vi "TCL.vi"() -> ()   [LabVIEW 2010]
uses:
  TPS Global.vi
panel:
  out "discarded fragments":string[](array[string])
  out "signals":cluster{"name":string, "values":string[]}[](array[cluster])
  out "events (last 11)":string[][](array[string])
  out "fragments":string[](array[string])
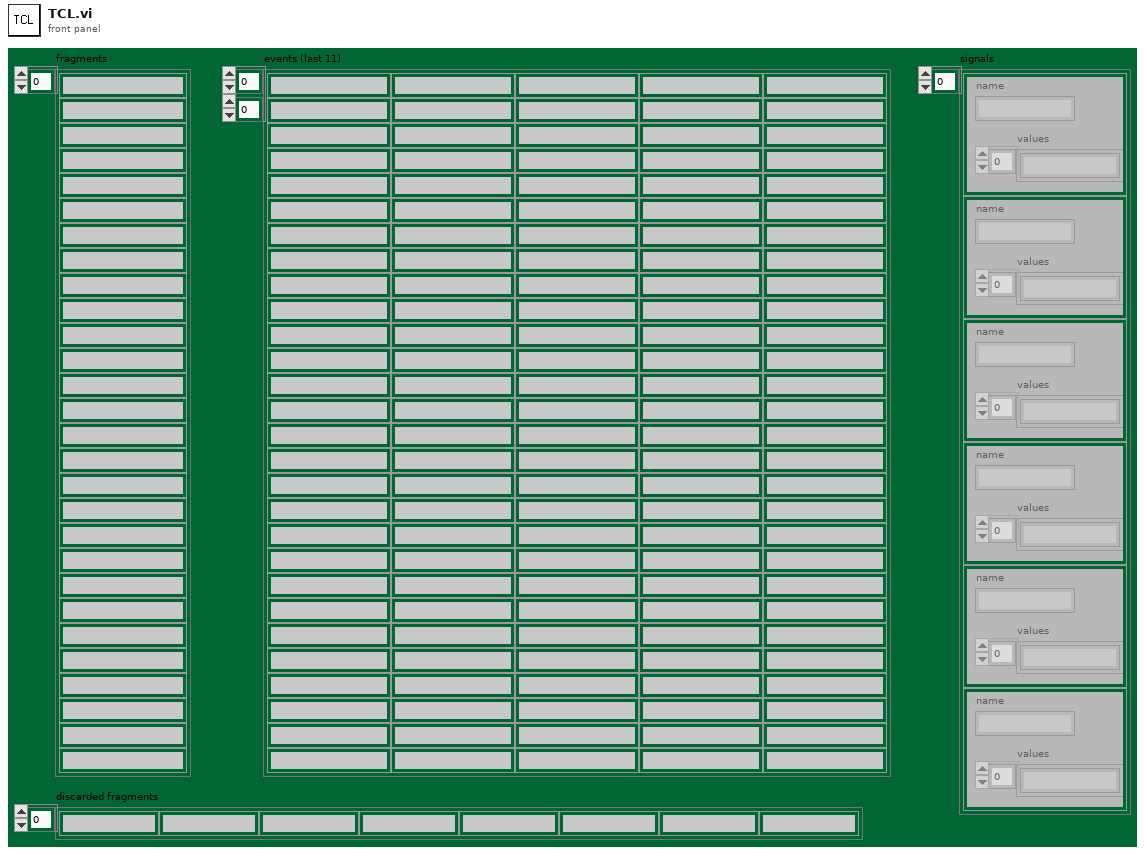
[diagram p1: front panel]
types:
  T1 = enum16{"open", "replace", "create", "open or create", "replace or create", "replace or create with confirmation"}
  T2 = enum16{"No Message", "Bad Message", "NewEventFile", "NewBaseFile", "Event=", "Ping=", "Address=", "Stop"}
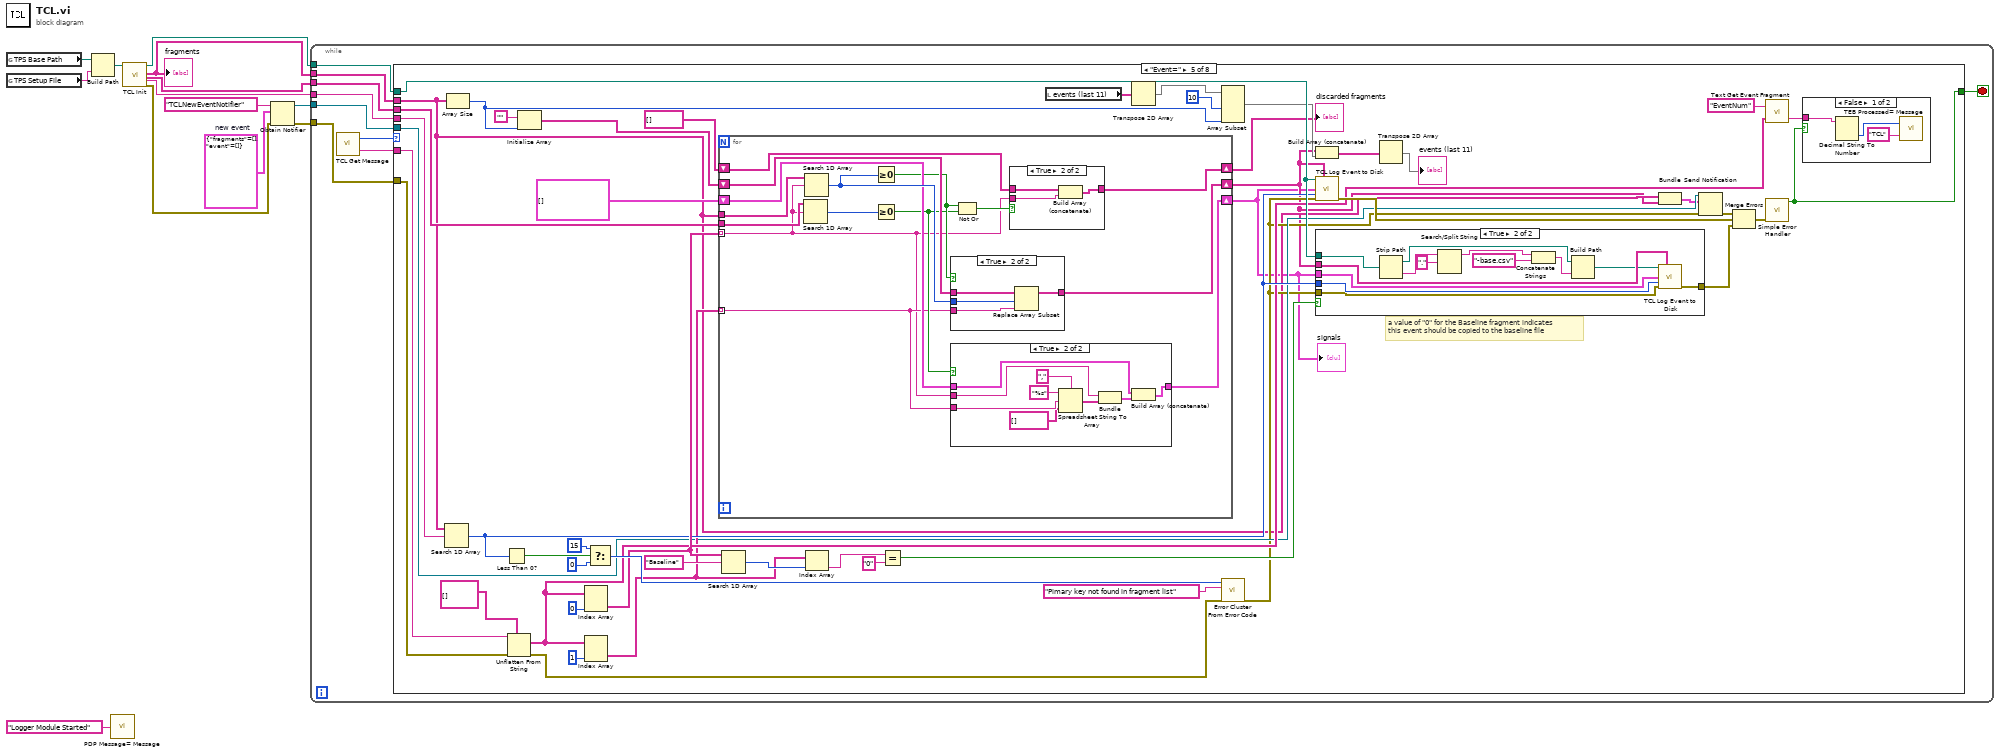
[diagram p0: block diagram]
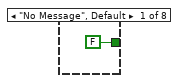
[diagram p2: hidden frame]
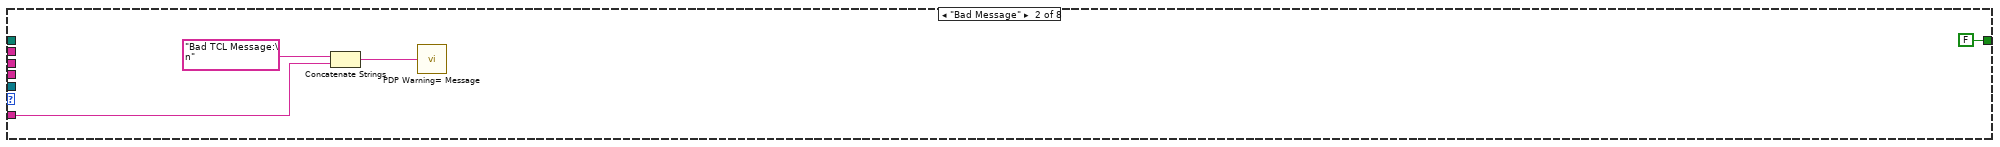
[diagram p3: hidden frame]
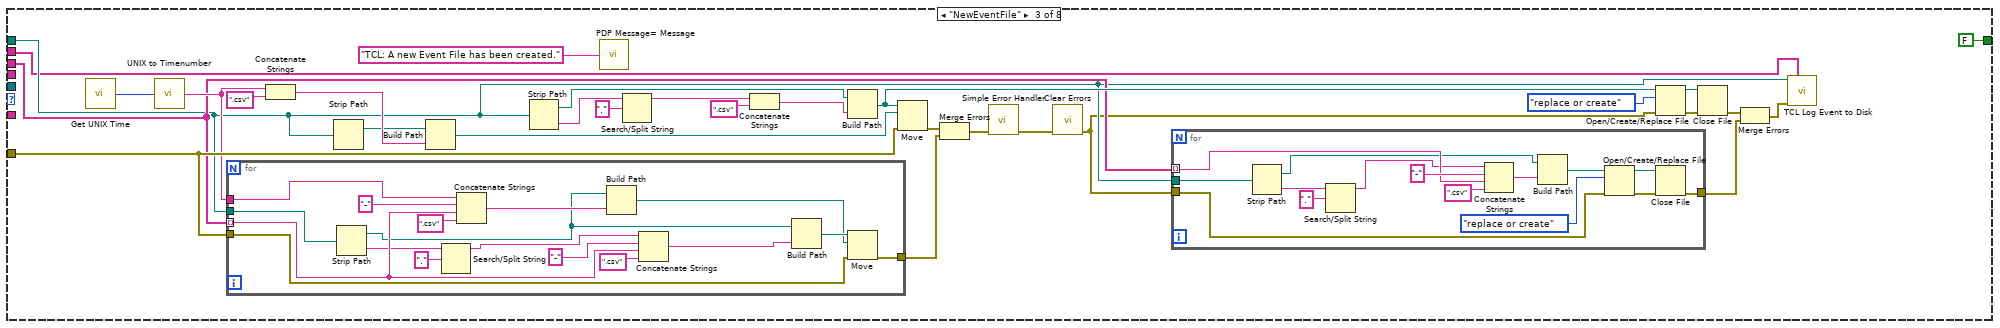
[diagram p4: hidden frame]
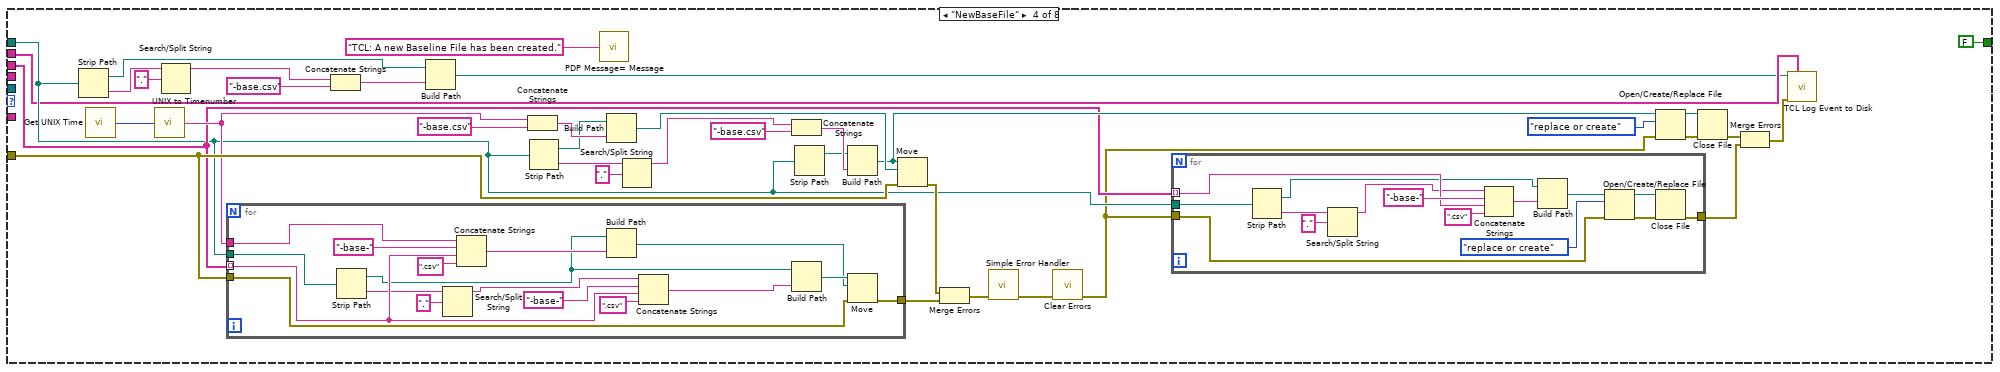
[diagram p5: hidden frame]
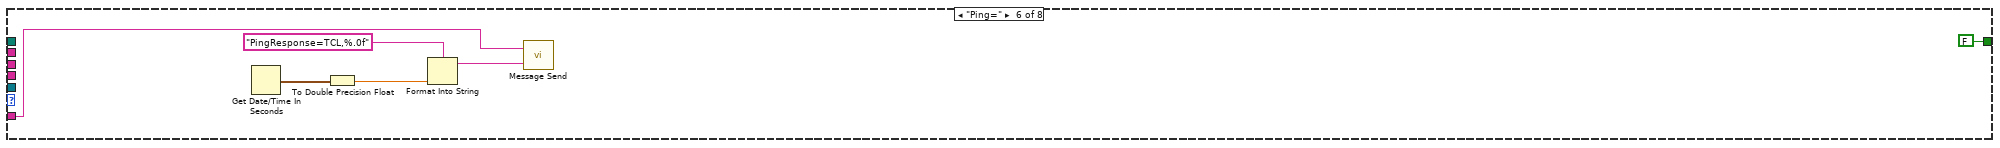
[diagram p11: hidden frame]
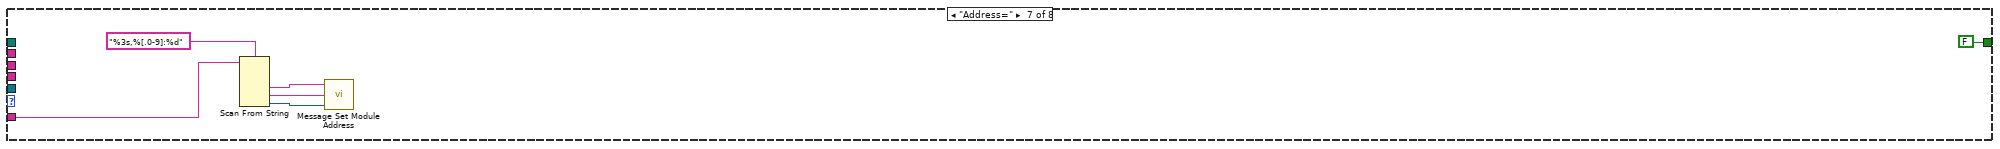
[diagram p12: hidden frame]
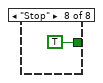
[diagram p13: hidden frame]
diagram:
  w3 = cluster{"fragments":string[], "event":string[]} {"fragments"=[], "event"=[]}  # new event
  n1 = global read "TPS Global.vi" "TPS Base Path"() -> (w12:path)
  n2 = global read "TPS Global.vi" "TPS Setup File"() -> (w11:string)
  n3 = Build Path(base path=w12, name or relative path=w11) -> (appended path=w10:path)
  n4 = call "PDP Message= Message.vi"("Message"="Logger Module Started") -> ()
  n5 = call "TCL Init.vi"("config file"=w10) -> ("event file"=w9:path, "fragments"=w6:string[], "signals"=w8:string[], "primary key"=w7:string, "error out"=w4:errorcluster)  [unwired: 14 in]
  "fragments" <- w6
  n6 = Obtain Notifier(name (unnamed)="TCLNewEventNotifier", notification data type=w3, error in (no error)=w4) -> (notifier out=w1:refnum<notifier>, error out=w5:errorcluster)  [unwired: 1 in, 1 out]
  n7 = while {
    tunnel: w5 -> [w20]
    tunnel: w9 -> [w19]
    tunnel: w8 -> [w18]
    tunnel: w6 -> [w17]
    tunnel: w7 -> [w15]
    tunnel: w1 -> [w14]
    stop <- w16 stop-if-true
    n8 = call "TCL Get Message.vi"() -> ("Text"=w21:string, "TCL Message Type"=w22:T2)
    n9 = case shown="\"Event=\"" w22 {
      tunnel: w21 -> [_ w25 _ _ w205 w259 w265 _]
      tunnel: w20 -> [_ _ w50 w119 w206 _ _ _]
      tunnel: w19 -> [_ _ w38 w107 w183 _ _ _]
      tunnel: w18 -> [_ _ w42 w111 w199 _ _ _]
      tunnel: w17 -> [_ _ w36 w105 w161 _ _ _]
      tunnel: [FALSE FALSE FALSE FALSE w167 FALSE FALSE TRUE] -> w16
      tunnel: w15 -> [_ _ _ _ w196 _ _ _]
      tunnel: w14 -> [_ _ _ _ w165 _ _ _]
      frame "No Message", Default {
      }
      frame "Bad Message" {
        n10 = Concatenate Strings("Bad TCL Message:\n" ("Message"), w25) -> (w26:string)
        n11 = call "PDP Warning= Message.vi"("Message"=w26) -> ()
      }
      frame "NewEventFile" {
        n12 = call "Get UNIX Time.vi"() -> ("UNIX seconds"=w56:i32)
        n13 = call "UNIX to Timenumber.vi"("Seconds"=w56) -> ("Timestamp String"=w49:string)
        n14 = for {
          tunnel: w42 -> [w79] mode=indexing
          tunnel: w50 -> [w89]
          tunnel: w38 -> [w83]
          tunnel: w49 -> [w80]
          tunnel: [w77] -> w48
          n15 = Strip Path(path=w83) -> (stripped path=w76:path, name=w73:string)
          n16 = Search/Split String(string=w73, search string/char (-)=".") -> (substring before match=w75:string)  [unwired: 1 in, 2 out]
          n17 = Concatenate Strings(w80, "-" ("string"), w79, ".csv" ("string")) -> (w82:string)
          n18 = Build Path(base path=w76, name or relative path=w82) -> (appended path=w84:path)
          n19 = Concatenate Strings(w75, "-" ("string"), w79, ".csv" ("string")) -> (w88:string)
          n20 = Build Path(base path=w76, name or relative path=w88) -> (appended path=w85:path)
          n21 = Move(source path=w85, error in=w89, 10:w84) -> (error out=w77:errorcluster)  [unwired: 2 in, 2 out]
        }
        n22 = Concatenate Strings(w49, ".csv" ("string")) -> (w52:string)
        n23 = Strip Path(path=w38) -> (stripped path=w32:path)  [unwired: 1 out]
        n24 = Build Path(base path=w32, name or relative path=w52) -> (appended path=w51:path)
        n25 = Strip Path(path=w38) -> (stripped path=w31:path, name=w28:string)
        n26 = call "PDP Message= Message.vi"("Message"="TCL: A new Event File has been created.") -> ()
        n27 = Search/Split String(string=w28, search string/char (-)=".") -> (substring before match=w30:string)  [unwired: 1 in, 2 out]
        n28 = Concatenate Strings(w30, ".csv" ("string")) -> (w54:string)
        n29 = Build Path(base path=w31, name or relative path=w54) -> (appended path=w45:path)
        n30 = Move(source path=w45, error in=w50, 10:w51) -> (error out=w47:errorcluster)  [unwired: 2 in, 2 out]
        n31 = Merge Errors(w47, w48) -> (w35:errorcluster)
        n32 = call <vilib>:"Simple Error Handler.vi"("error in (no error)"=w35) -> ("error out"=w34:errorcluster)  [unwired: 4 in, 4 out]
        n33 = call <vilib>:"Clear Errors.vi"("error in (no error)"=w34) -> ("error out"=w33:errorcluster)  [unwired: 6 in]
        n34 = for {
          tunnel: w42 -> [w70] mode=indexing
          tunnel: w38 -> [w68]
          tunnel: w33 -> [w66]
          tunnel: [w62] -> w41
          n35 = Strip Path(path=w68) -> (stripped path=w61:path, name=w59:string)
          n36 = Search/Split String(string=w59, search string/char (-)=".") -> (substring before match=w58:string)  [unwired: 1 in, 2 out]
          n37 = Concatenate Strings(w58, "-" ("string"), w70, ".csv" ("string")) -> (w69:string)
          n38 = Build Path(base path=w61, name or relative path=w69) -> (appended path=w67:path)
          n39 = Open/Create/Replace File(file path (use dialog)=w67, error in=w66, operation (0:open)=T1."replace or create") -> (refnum out=w64:refnum<file>, error out=w63:errorcluster)  [unwired: 3 in, 1 out]
          n40 = Close File(refnum=w64, error in=w63) -> (error out=w62:errorcluster)  [unwired: 1 out]
        }
        n41 = Open/Create/Replace File(file path (use dialog)=w45, error in=w33, operation (0:open)=T1."replace or create") -> (refnum out=w44:refnum<file>, error out=w43:errorcluster)  [unwired: 3 in, 1 out]
        n42 = Close File(refnum=w44, error in=w43) -> (error out=w40:errorcluster)  [unwired: 1 out]
        n43 = Merge Errors(w40, w41) -> (w39:errorcluster)
        n44 = call "TCL Log Event to Disk.vi"("event file"=w38, "event"=w36, "error in (no error)"=w39) -> ()  [unwired: 12 in, 1 out]
      }
      frame "NewBaseFile" {
        n45 = Strip Path(path=w107) -> (stripped path=w95:path, name=w91:string)
        n46 = call "Get UNIX Time.vi"() -> ("UNIX seconds"=w125:i32)
        n47 = call "UNIX to Timenumber.vi"("Seconds"=w125) -> ("Timestamp String"=w118:string)
        n48 = Search/Split String(string=w91, search string/char (-)=".") -> (substring before match=w92:string)  [unwired: 1 in, 2 out]
        n49 = for {
          tunnel: w111 -> [w148] mode=indexing
          tunnel: w119 -> [w158]
          tunnel: w107 -> [w152]
          tunnel: w118 -> [w149]
          tunnel: [w146] -> w117
          n50 = Strip Path(path=w152) -> (stripped path=w145:path, name=w143:string)
          n51 = Search/Split String(string=w143, search string/char (-)=".") -> (substring before match=w142:string)  [unwired: 1 in, 2 out]
          n52 = Concatenate Strings(w149, "-base-" ("string"), w148, ".csv" ("string")) -> (w151:string)
          n53 = Build Path(base path=w145, name or relative path=w151) -> (appended path=w153:path)
          n54 = Concatenate Strings(w142, "-base-" ("string"), w148, ".csv" ("string")) -> (w157:string)
          n55 = Build Path(base path=w145, name or relative path=w157) -> (appended path=w154:path)
          n56 = Move(source path=w154, error in=w158, 10:w153) -> (error out=w146:errorcluster)  [unwired: 2 in, 2 out]
        }
        n57 = Concatenate Strings(w92, "-base.csv" ("string")) -> (w93:string)
        n58 = Build Path(base path=w95, name or relative path=w93) -> (appended path=w94:path)
        n59 = Concatenate Strings(w118, "-base.csv" ("string")) -> (w121:string)
        n60 = Strip Path(path=w107) -> (stripped path=w100:path, name=w98:string)
        n61 = call "PDP Message= Message.vi"("Message"="TCL: A new Baseline File has been created.") -> ()
        n62 = Build Path(base path=w100, name or relative path=w121) -> (appended path=w120:path)
        n63 = Search/Split String(string=w98, search string/char (-)=".") -> (substring before match=w96:string)  [unwired: 1 in, 2 out]
        n64 = Concatenate Strings(w96, "-base.csv" ("string")) -> (w123:string)
        n65 = Strip Path(path=w107) -> (stripped path=w99:path)  [unwired: 1 out]
        n66 = Build Path(base path=w99, name or relative path=w123) -> (appended path=w114:path)
        n67 = Move(source path=w114, error in=w119, 10:w120) -> (error out=w116:errorcluster)  [unwired: 2 in, 2 out]
        n68 = Merge Errors(w116, w117) -> (w103:errorcluster)
        n69 = call <vilib>:"Simple Error Handler.vi"("error in (no error)"=w103) -> ("error out"=w102:errorcluster)  [unwired: 4 in, 4 out]
        n70 = call <vilib>:"Clear Errors.vi"("error in (no error)"=w102) -> ("error out"=w101:errorcluster)  [unwired: 6 in]
        n71 = for {
          tunnel: w111 -> [w139] mode=indexing
          tunnel: w107 -> [w137]
          tunnel: w101 -> [w135]
          tunnel: [w131] -> w110
          n72 = Strip Path(path=w137) -> (stripped path=w130:path, name=w128:string)
          n73 = Search/Split String(string=w128, search string/char (-)=".") -> (substring before match=w127:string)  [unwired: 1 in, 2 out]
          n74 = Concatenate Strings(w127, "-base-" ("string"), w139, ".csv" ("string")) -> (w138:string)
          n75 = Build Path(base path=w130, name or relative path=w138) -> (appended path=w136:path)
          n76 = Open/Create/Replace File(file path (use dialog)=w136, error in=w135, operation (0:open)=T1."replace or create") -> (refnum out=w133:refnum<file>, error out=w132:errorcluster)  [unwired: 3 in, 1 out]
          n77 = Close File(refnum=w133, error in=w132) -> (error out=w131:errorcluster)  [unwired: 1 out]
        }
        n78 = Open/Create/Replace File(file path (use dialog)=w114, error in=w101, operation (0:open)=T1."replace or create") -> (refnum out=w113:refnum<file>, error out=w112:errorcluster)  [unwired: 3 in, 1 out]
        n79 = Close File(refnum=w113, error in=w112) -> (error out=w109:errorcluster)  [unwired: 1 out]
        n80 = Merge Errors(w109, w110) -> (w108:errorcluster)
        n81 = call "TCL Log Event to Disk.vi"("event file"=w94, "event"=w105, "error in (no error)"=w108) -> ()  [unwired: 12 in, 1 out]
      }
      frame "Event=" {
        # "a value of \"0\" for the Baseline fragment indicates\nthis event should be copied to the baseline file"
        n82 = Search 1D Array(1D array=w161, element=w196) -> (index of element=w182:i32)  [unwired: 1 in]
        n83 = Array Size(array=w161) -> (size(s)=w172:i32)
        n84 = Less Than 0?(x=w182) -> (x < 0?=w193:bool)
        n85 = Unflatten From String(type=string[][] [], binary string=w205, error in (no error)=w206) -> (value=w176:string[][], error out=w195:errorcluster)  [unwired: 2 in, 1 out]
        n86 = Initialize Array("", w172) -> (w201:string[])
        n87 = Index Array(array=w176, index (col)=0) -> (element=w189:string[])  [unwired: 1 in]
        n88 = Index Array(array=w176, index (col)=1) -> (element=w166:string[])  [unwired: 1 in]
        n89 = Select(t=15, s=w193, f=0) -> (s? t:f=w192:i32)
        n90 = for {
          tunnel: w189 -> [w224] mode=indexing
          tunnel: w166 -> [w226] mode=indexing
          tunnel: w161 -> [w238]
          tunnel: w199 -> [w237]
          shift-right: [w234] -> w160
          shift-left: w201 -> [w235]
          shift-right: [w225] -> w170
          shift-left: string[] [] -> [w227]
          shift-right: [w231] -> w159
          shift-left: cluster{"name":string, "values":string[]}[] [] ("signals") -> [w232]
          n91 = Search 1D Array(1D array=w237, element=w224) -> (index of element=w233:i32)  [unwired: 1 in]
          n92 = Search 1D Array(1D array=w238, element=w224) -> (index of element=w236:i32)  [unwired: 1 in]
          n93 = Greater Or Equal To 0?(x=w236) -> (x >= 0?=w230:bool)
          n94 = Greater Or Equal To 0?(x=w233) -> (x >= 0?=w229:bool)
          n95 = case shown="True" w230 {
            tunnel: w236 -> [_ w257]
            tunnel: w226 -> [_ w256]
            tunnel: w235 -> [w253 w255]
            tunnel: [w253 w254] -> w234
            frame False {
            }
            frame True {
              n96 = Replace Array Subset(array=w255, new element=w256, index=w257) -> (w254:string[])
            }
          }
          n97 = case shown="True" w229 {
            tunnel: w232 -> [w243 w252]
            tunnel: w224 -> [_ w250]
            tunnel: w226 -> [_ w247]
            tunnel: [w243 w244] -> w231
            frame False {
            }
            frame True {
              n98 = Spreadsheet String To Array(delimiter (Tab)=",", format string="%s", spreadsheet string=w247, array type (2D Dbl)=string[] []) -> (array=w246:string[])
              n99 = Bundle(w250, w246) -> (w251:cluster{string, string[]})  [unwired: 1 in]
              n100 = Build Array (concatenate)(w252, w251) -> (w244:cluster{"name":string, "values":string[]}[])
            }
          }
          n101 = Not Or(1:w229, 2:w230) -> (0:w228:bool)
          n102 = case shown="True" w228 {
            tunnel: w227 -> [w239 w242]
            tunnel: w224 -> [_ w241]
            tunnel: [w239 w240] -> w225
            frame False {
            }
            frame True {
              n103 = Build Array (concatenate)(w242, w241) -> (w240:string[])
            }
          }
        }
        "discarded fragments" <- w170
        "signals" <- w159
        n104 = Search 1D Array(1D array=w189, element="Baseline") -> (index of element=w187:i32)  [unwired: 1 in]
        n105 = Index Array(array=w166, index=w187) -> (element=w186:string)
        n106 = Equal?(x=w186, y="0") -> (x = y?=w184:bool)
        n107 = local read "events (last 11)"() -> (w168:string[][])
        n108 = Transpose 2D Array(2D array=w168) -> (transposed array=w171:string[][])
        n109 = Array Subset(array=w171, length (row)=10, length (col)=w172) -> (w173:string[][])  [unwired: 2 in]
        n110 = call <vilib>:"Error Cluster From Error Code.vi"("error in (no error)"=w195, "error message (\"\")"="Pimary key not found in fragment list" ("error message (\"\")"), "error code (0)"=w192) -> ("error out"=w164:errorcluster)  [unwired: 6 in]
        n111 = Build Array (concatenate)(w160, w173) -> (w174:string[][])
        n112 = call "TCL Log Event to Disk.vi"("event file"=w183, "event"=w160, "signals"=w159, "primary key"=w182, "error in (no error)"=w164) -> ("error out"=w181:errorcluster)  [unwired: 10 in]
        n113 = case shown="True" w184 {
          tunnel: w160 -> [_ w223]
          tunnel: w183 -> [_ w222]
          tunnel: w159 -> [_ w220]
          tunnel: w182 -> [_ w219]
          tunnel: w164 -> [w210 w218]
          tunnel: [w210 w217] -> w180
          frame False {
          }
          frame True {
            n114 = Strip Path(path=w222) -> (stripped path=w213:path, name=w216:string)
            n115 = Search/Split String(string=w216, search string/char (-)=".") -> (substring before match=w214:string)  [unwired: 1 in, 2 out]
            n116 = Concatenate Strings(w214, "-base.csv" ("string")) -> (w211:string)
            n117 = Build Path(base path=w213, name or relative path=w211) -> (appended path=w212:path)
            n118 = call "TCL Log Event to Disk.vi"("event file"=w212, "event"=w223, "signals"=w220, "primary key"=w219, "error in (no error)"=w218) -> ("error out"=w217:errorcluster)  [unwired: 10 in]
          }
        }
        n119 = Transpose 2D Array(2D array=w174) -> (transposed array=→"events (last 11)":string[][])
        n120 = Bundle("fragments"=w161, w160) -> (w162:cluster{"fragments":string[], string[]})  [unwired: 1 in]
        n121 = Send Notification(notification=w162, notifier=w165, error in (no error)=w164) -> (error out=w163:errorcluster)  [unwired: 1 out]
        n122 = Merge Errors(w163, w181, w180) -> (w179:errorcluster)
        n123 = call "Text Get Event Fragment.vi"("Event"=w176, "Fragment Type"="EventNum") -> ("Fragment"=w177:string)  [unwired: 1 out]
        n124 = call <vilib>:"Simple Error Handler.vi"("error in (no error)"=w179) -> ("error?"=w167:bool)  [unwired: 4 in, 4 out]
        n125 = case shown="False" w167 {
          tunnel: w177 -> [w207 _]
          frame False {
            n126 = Decimal String To Number(string=w207) -> (number=w208:i32)  [unwired: 2 in, 1 out]
            n127 = call "TEB Processed= Message.vi"("Module Name"="TCL", "Event Number"=w208) -> ()
          }
          frame True {
          }
        }
      }
      frame "Ping=" {
        n128 = Get Date/Time In Seconds() -> (seconds since 1Jan1904=w260:timestamp)
        n129 = To Double Precision Float(number=w260) -> (double precision float=w262:dbl)
        n130 = Format Into String(format string="PingResponse=TCL,%.0f", w262) -> (resulting string=w261:string)  [unwired: 2 in, 1 out]
        n131 = call "Message Send.vi"("Message"=w261, "Destination"=w259) -> ()
      }
      frame "Address=" {
        n132 = Scan From String(format string="%3s,%[.0-9]:%d" ("Format String"), input string=w265) -> (output 1=w267:string, output 2=w268:string, output 3=w266:i32)  [unwired: 5 in, 3 out]
        n133 = call "Message Set Module Address.vi"("Port"=w266, "Address"=w268, "Module"=w267) -> ()
      }
      frame "Stop" {
      }
    }
  }
